vi "Init SequenceCountService.vi"(8 "error in (no error)":errorcluster, 11 "Vecto in":refnum<class "Vecto.lvclass">) -> (0 "error out":errorcluster, 3 "Vecto out":refnum<class "Vecto.lvclass">)   [LabVIEW 2020, in "Vecto.lvlib" / "Vecto.lvclass"]
uses:
  Vecto.lvclass
  Vecto.lvclass/Vecto.ctl
  SequenceCountService/SequenceCountService.lvclass
  C:/dev/lv20CE/lv-vecto/Vecto/Service/Service.lvclass
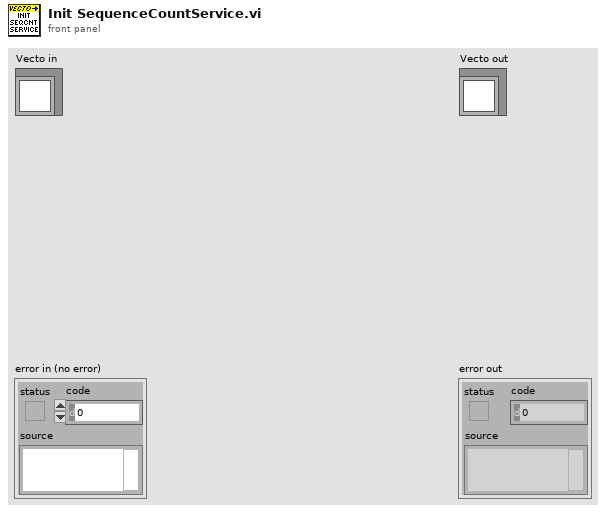
[diagram p1: front panel]
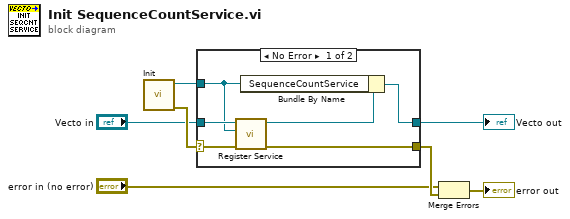
[diagram p0: block diagram]
diagram:
  n1 = call "Init.vi"() -> ("error out"=w7:errorcluster, "SequenceCountService out"=w5:refnum<class "SequenceCountService.lvclass">)  [unwired: 10 in]
  n2 = case shown="No Error" w7 {
    selector: w7 -> [w13 w14]
    tunnel: "Vecto in" -> [w12 w15]
    tunnel: w5 -> [w10 _]
    tunnel: [w9 w15] -> w1
    tunnel: [w8 w14] -> w4
    frame No Error {
      n3 = call "Register Service.vi"("error in (no error)"=w13, "Service"=w10, "Vecto in"=w12) -> ("error out"=w8:errorcluster, "Vecto out"=w11:refnum<class "Vecto.lvclass">)  [unwired: 7 in]
      n4 = Bundle By Name(cluster=w11, "SequenceCountService"=w10) -> (w9:refnum<class "Vecto.lvclass">)
    }
    frame Error {
    }
  }
  "Vecto out" <- w1
  n5 = Merge Errors("error in (no error)", w4) -> (→"error out":errorcluster)
